vi "Y_profile.vi"(2 "no. of lines until end of fly-back":u16, 3 "line counter":u16, 4 "no. of lines until start of fly-back":u16, 5 "y amplitude":u16, 6 "y step size":u16, 7 "true when line counter smaller than y resolution":bool) -> (0 "y signal":i16)   [LabVIEW 2010]
panel:
  out "coerced(x)":u16
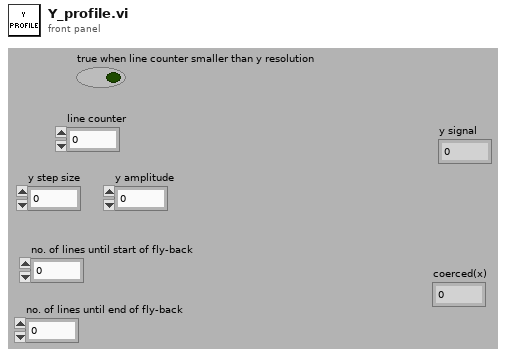
[diagram p1: front panel]
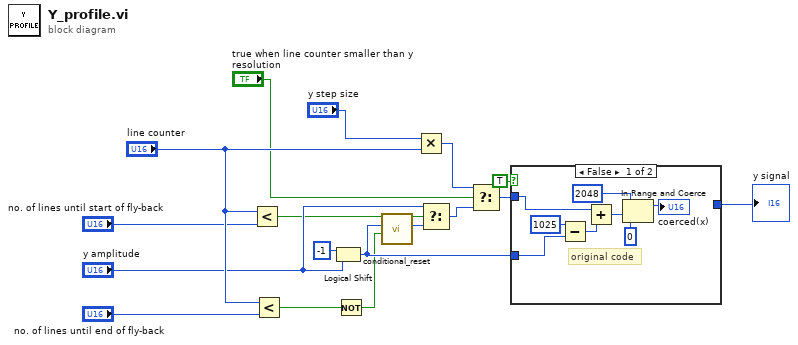
[diagram p0: block diagram]
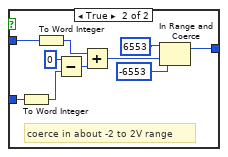
[diagram p2: hidden frame]
diagram:
  n1 = Less?(x="line counter", y="no. of lines until start of fly-back") -> (x < y?=w2:bool)
  n2 = Less?(x="line counter", y="no. of lines until end of fly-back") -> (x < y?=w5:bool)
  n3 = Logical Shift(y=i16 -1 ("n"), x="y amplitude") -> (x << y=w15:u16)
  n4 = Not(x=w5) -> (.not. x?=w13:bool)
  n5 = call "conditional_reset.vi"("reset?"=w13, "number in"=w15) -> ("number out"=w6:u16)  [unwired: 4 in]
  n6 = Multiply(x="y step size", y="line counter") -> (x*y=w3:u16)
  n7 = Select(t="y amplitude", s=w2, f=w6) -> (s? t:f=w11:u16)
  n8 = Select(t=w3, s="true when line counter smaller than y resolution", f=w11) -> (s? t:f=w9:u16)
  n9 = case shown="False" TRUE {
    tunnel: [_ w28] -> w7
    tunnel: w15 -> [w19 w26]
    tunnel: w9 -> [w20 w27]
    frame False {
      # "original code"
      n10 = Subtract(x=u16 1025, y=w19) -> (x-y=w22:u16)
      n11 = Add(x=w20, y=w22) -> (x+y=w21:u16)
      n12 = In Range and Coerce(upper limit=u16 2048, x=w21, lower limit=u16 0) -> (coerced(x)=→"coerced(x)":u16)  [unwired: 1 out]
    }
    frame True {
      # "coerce in about -2 to 2V range"
      n13 = To Word Integer(number=w26) -> (16bit integer=w33:i16)
      n14 = To Word Integer(number=w27) -> (16bit integer=w32:i16)
      n15 = Subtract(x=i16 0, y=w33) -> (x-y=w34:i16)
      n16 = Add(x=w32, y=w34) -> (x+y=w29:i16)
      n17 = In Range and Coerce(upper limit=i16 6553, x=w29, lower limit=i16 -6553) -> (coerced(x)=w28:i16)  [unwired: 1 out]
    }
  }
  "y signal" <- w7
